vi "Do.vi"(8 "error in (no error)":errorcluster, 10 "Actor in":refnum<class "Actor.lvclass">, 11 "Yokogawa Class Chooser Msg":refnum<class "Yokogawa Class Chooser Msg.lvclass">) -> (0 "error out":errorcluster, 2 "Actor out":refnum<class "Actor.lvclass">)   [LabVIEW 2013, in "Universal Power Meter.lvlib" / "Yokogawa Class Chooser Msg.lvclass"]
doc: "This VI delivers the message to the actor by calling the appropriate method(s) on the actor."
uses:
  Yokogawa Class Chooser Msg.lvclass
  <vilib>/ActorFramework/Actor/Actor.lvclass
  Yokogawa Class Chooser Msg.lvclass/Yokogawa Class Chooser Msg.ctl
  Universal Power Meter class/Universal Power Meter.lvclass
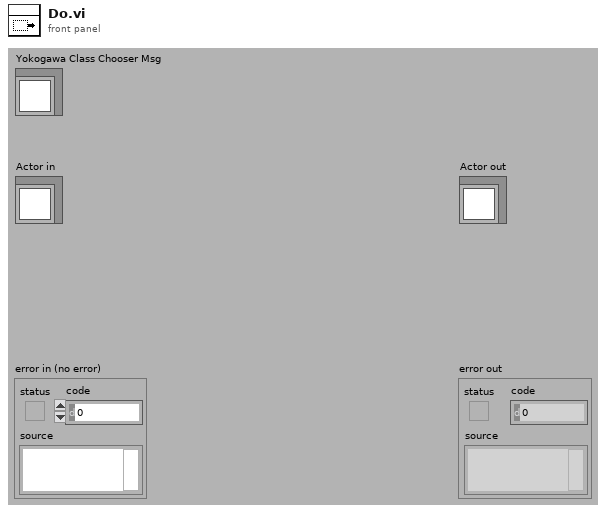
[diagram p1: front panel]
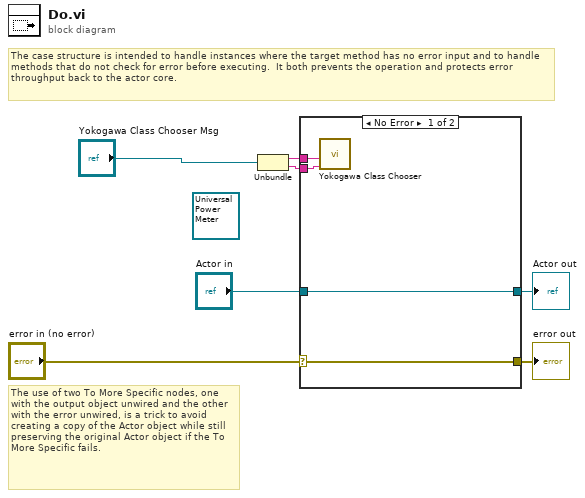
[diagram p0: block diagram]
diagram:
  (unwired) refnum<class "Universal Power Meter.lvclass"> refnum ("Actor in")
  # "The use of two To More Specific nodes, one with the output object unwired and the other with the error unwired, is a trick to avoid creating a copy of the Actor object while still preserving the original Actor object if the To More Specific fails."
  # "The case structure is intended to handle instances where the target method has no error input and to handle methods that do not check for error before executing.  It both prevents the operation and protects error throughput back to the actor core."
  n1 = Unbundle("Yokogawa Class Chooser Msg") -> (w3:string, w1:string)
  n2 = case shown="No Error" "error in (no error)" {
    selector: "error in (no error)" -> [w11 w13]
    tunnel: [w11 w13] -> w6
    tunnel: [w9 w12] -> w5
    tunnel: "Actor in" -> [w9 w12]
    tunnel: w3 -> [w10 _]
    tunnel: w1 -> [w8 _]
    frame No Error {
      n3 = call "Yokogawa Class Chooser.vi"("Incoming Otpion"=w8, "Incoming ID"=w10) -> ()  [unwired: 9 in, 1 out]
    }
    frame Error {
      # "If type check fails, pass the original object out again."
    }
  }
  "error out" <- w6
  "Actor out" <- w5
